vi "Requests.vi"(8 "error in (no error)":errorcluster, 9 "write enable":bool=TRUE, 11 "ICPCON ET-7018 in":refnum<class "ICPCON ET-7024i.lvclass">) -> (0 "error out":errorcluster, 3 "ICPCON ET-7018 out":refnum<class "ICPCON ET-7024i.lvclass">)   [LabVIEW 2021, in "ICPCON ET-7024i.lvclass"]
uses:
  ICPCON ET-7024i.lvclass
  D:/my_projects/projects/Algorithms/Labview/21/Modbus/MB_TCP2/MB_TCP.lvclass
  MB_TCP.lvclass/MB_TCP.ctl
  NI_modbus_upd/Ctl/Unit_ID.ctl
  NI_modbus_upd/TCP/TCP.lvclass/TCP.ctl
  NI_modbus_upd/Master Function Definition/Responses/Read Discrete Inputs Response.vi
  NI_modbus_upd/Master network read write.vi
  NI_modbus_upd/Master Function Definition/Requests/Read Discrete Inputs Request.vi
  NI_modbus_upd/Master Function Definition/Responses/Read Coils Response.vi
  NI_modbus_upd/Master Function Definition/Requests/Read Coils Request.vi
  NI_modbus_upd/Master Function Definition/Responses/Read Holding Registers Response.vi
  NI_modbus_upd/Master Function Definition/Requests/Read Holding Registers Request.vi
  NI_modbus_upd/Utility/Bytes to Bits1.vi
  NI_modbus_upd/Function code mismatch error1.vi
  NI_modbus_upd/Error Generator1.vi
  NI_modbus_upd/Read ADU Packet Master.vi
  NI_modbus_upd/Write ADU Packet Master.vi
  NI_modbus_upd/Modbus Data Unit (PDU)/Construct PDU1.vi
  NI_modbus_upd/Utility/Bytes to U16s1.vi
  NI_modbus_upd/Modbus Data Unit (PDU)/Unflatten to PDU1.vi
  NI_modbus_upd/TCP/Protocol Read.vi
  NI_modbus_upd/TCP/Protocol Write.vi
  <vilib>/Utility/error.llb/Clear Errors.vi
  NI_modbus_upd/Modbus Data Unit (PDU)/Deconstruct PDU1.vi
  NI_modbus_upd/TCP/TCP.lvclass
  ICPCON Registers/ICPCON Registers.lvlib
  MB_TCP.lvclass
  NI_modbus_upd/NI_modbus_upd.lvlib
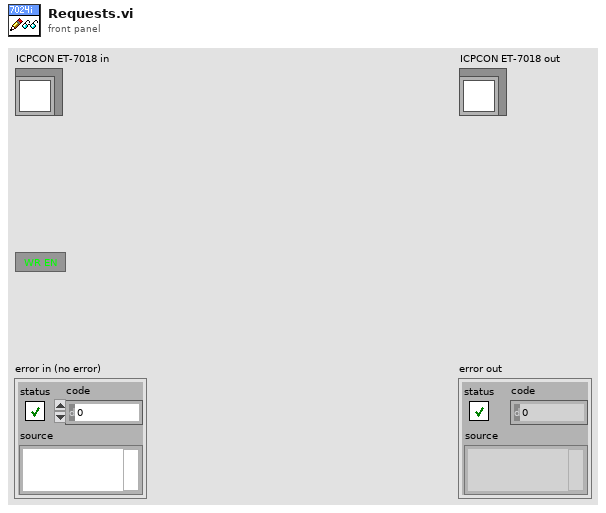
[diagram p1: front panel]
types:
  T1 = typedef "NI_modbus_upd.lvlib/Unit_ID.ctl" = cluster{"Protocol ID":u16, "Unit ID":u8}
  T2 = typedef "ICPCON Registers.lvlib/ICPCON Data.ctl" = cluster{"UTF":refnum<data-value>, "DI":refnum<data-value>, "DW":refnum<data-value>, "DO":refnum<data-value>, "IR":refnum<data-value>, "WR":refnum<data-value>, "OR":refnum<data-value>, "modified":refnum<data-value>}
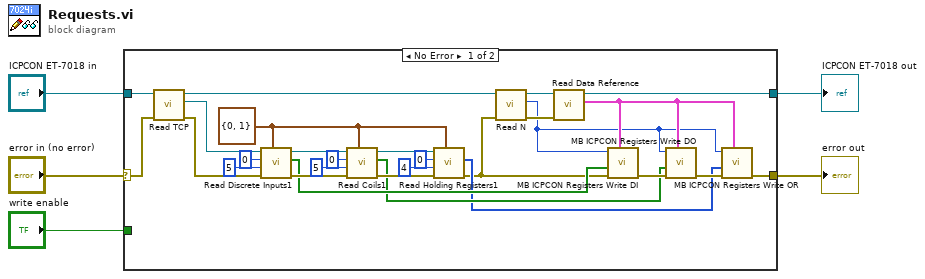
[diagram p0: block diagram]
diagram:
  n1 = case shown="No Error" "error in (no error)" {
    selector: "error in (no error)" -> [w8 w35]
    tunnel: [w31 w35] -> w3
    tunnel: [w6 w34] -> w4
    tunnel: "ICPCON ET-7018 in" -> [w9 w34]
    tunnel: "write enable" -> [_ _]
    frame No Error {
      w13 = T1 {"Protocol ID"=0, "Unit ID"=1} ("Unit_ID")
      n2 = call "Read TCP.vi"("error in (no error)"=w8, "MB_TCP in"=w9) -> ("error out"=w16:errorcluster, "TCP"=w18:refnum<class "TCP.lvclass">, "MB_TCP out"=w17:refnum<class "ICPCON ET-7024i.lvclass">)  [unwired: 7 in]
      n3 = call "Read Discrete Inputs1.vi"("Unit_ID"=w13, "error in (no error)"=w16, "number of discrete inputs"=u16 5, "starting address"=u16 0, "Modbus master in"=w18) -> ("error out"=w19:errorcluster, "discrete input values"=w12:bool[], "Modbus master out"=w15:refnum<class "TCP.lvclass">)  [unwired: 4 in]
      n4 = call "Read Coils1.vi"("Unit_ID"=w13, "error in (no error)"=w19, "number of coils"=u16 5 ("number of discrete inputs"), "starting address"=u16 0, "Modbus master in"=w15) -> ("error out"=w22:errorcluster, "coil values"=w11:bool[], "Modbus master out"=w14:refnum<class "TCP.lvclass">)  [unwired: 4 in]
      n5 = call "Read Holding Registers1.vi"("Unit_ID"=w13, "error in (no error)"=w22, "number of holding registers"=u16 4 ("number of discrete inputs"), "starting address"=u16 0, "Modbus master in"=w14) -> ("error out"=w7:errorcluster, "register values"=w10:u16[])  [unwired: 4 in, 1 out]
      n6 = call "Read N.vi"("error in (no error)"=w7, "MB_TCP in"=w17) -> ("error out"=w29:errorcluster, "N"=w27:i32, "MB_TCP out"=w30:refnum<class "ICPCON ET-7024i.lvclass">)  [unwired: 7 in]
      n7 = call "Read Data Reference.vi"("error in (no error)"=w29, "MB_TCP in"=w30) -> ("Data"=w28:T2, "MB_TCP out"=w6:refnum<class "ICPCON ET-7024i.lvclass">)  [unwired: 7 in, 1 out]
      n8 = call "MB ICPCON Registers Write DI.vi"("Data Reference"=w28, "error in (no error)"=w7, "Bits In"=w12, "N"=w27) -> ("error out"=w33:errorcluster)  [unwired: 7 in]
      n9 = call "MB ICPCON Registers Write DO.vi"("Data Reference"=w28, "error in (no error)"=w33, "Bits In"=w11, "N"=w27) -> ("error out"=w32:errorcluster)  [unwired: 7 in]
      n10 = call "MB ICPCON Registers Write OR.vi"("Data Reference"=w28, "error in (no error)"=w32, "Words In"=w10, "N"=w27) -> ("error out"=w31:errorcluster)  [unwired: 7 in]
    }
    frame Error {
    }
  }
  "error out" <- w3
  "ICPCON ET-7018 out" <- w4
